vi "标定程序.vi"() -> ()   [LabVIEW 2016]
uses:
  <vilib>/userdefined/High Color/IMAQdx.ctl
  <vilib>/vision/driver/IMAQdx.llb/IMAQdx Acquisition Mode.ctl
  <vilib>/vision/driver/IMAQdx.llb/IMAQdx Buffer Number Mode.ctl
  <vilib>/Utility/config.llb/Read Key (Double).vi
  <vilib>/vision/driver/NI_Vision_Acquisition_Software.lvlib
  <vilib>/Utility/config.llb/NI_LVConfig.lvlib
panel:
  out "Top":cluster{"下边缘设置：":i32, "右边缘设置：":i32}
  out "Bottom":cluster{"上边缘设置：":i32, "右边缘设置：":i32}
  out "CamAng":dbl
  out "RobAng":dbl
  in  "选项卡控件":enum32{"选项卡 1"}(tab)
  out "Image":T1(plugin-control)
  out "机械手参数设置":bool
  out "机械手连接":bool
  out "相机一次采集":bool
  out "机械手X轴移动":bool
  out "相机二次采集":bool
  out "示教圆心":bool
  out "参数保存":bool
  in  "机械手IP地址":string="10.193.13.22"
  in  "机械手端口号":string="54600"
  in  "X轴偏移量":string="10"
  in  "Y轴偏移量":string="10"
  out "机械手Y轴移动":bool
  out "相机三次采集":bool
  in  "Fail步骤":string
  out "机械手当前X坐标":dbl
  out "机械手当前Y坐标":dbl
  out "圆心像素X坐标":dbl
  out "圆心像素Y坐标":dbl
  in  "确定按钮":bool
  in  "强制退出":bool
  out "停止2":bool
  out "停止":bool
  out "数组 2":dbl[](array[numeric])
  out "数组":dbl[](array[numeric])
  out "是否重建模板":bool
  in  "操作状态":string
  out "step8":bool
  out "step7":bool
  out "step6":bool
  out "step5":bool
  out "step4":bool
  out "step3":bool
  out "step2":bool
  out "执行状态":bool
  in  "机械手坐标系":string
  out "step1":bool
  # "库卡机械手视觉标定程序"
  # "V1.0"
  # "机械手参数显示"
  # "视觉影像显示"
  # "位置参数显示"
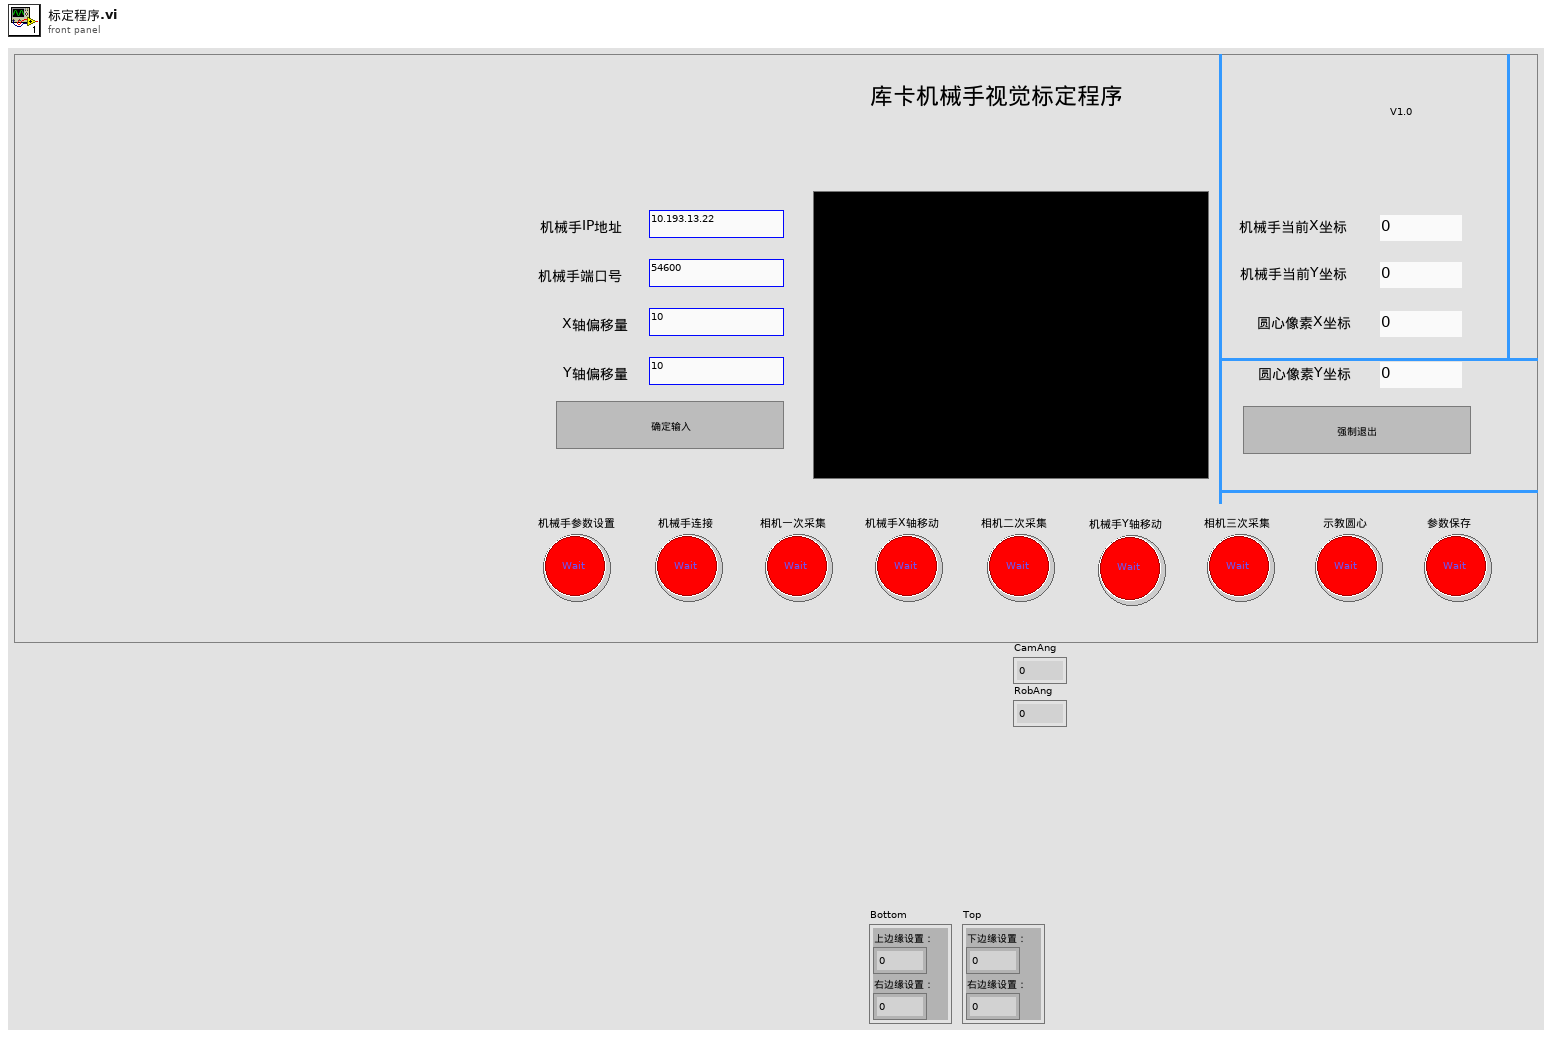
[diagram p1: front panel]
types:
  T1 = typedef "IMAQ Image.ctl" = refnum<image>
  T2 = typedef "NI_Vision_Acquisition_Software.lvlib/IMAQdx Acquisition Mode.ctl" = enum32{"One Shot", "Continuous"}
  T3 = typedef "IMAQdx.ctl" = refnum<k21>
  T4 = enum16{"初始化", "机械手参数设置", "机械手连接", "相机一次采集", "机械手X轴移动", "相机二次采集", "机械手Y轴移动", "相机三次采集", "示教基准位置", "保存参数", "完成"}
  T5 = enum16{"Standard", "Buffered", "CRLF", "Immediate"}
  T6 = typedef "NI_Vision_Acquisition_Software.lvlib/IMAQdx Buffer Number Mode.ctl" = enum32{"Next", "Last", "Buffer Number", "Every", "Last New"}
  T7 = enum32{"Invalid", "Standard", "Closed", "Hidden", "Minimized", "Maximized"}
  T8 = typedef "NI_LVConfig.lvlib/Config Data RefNum.ctl" = refnum<k1>
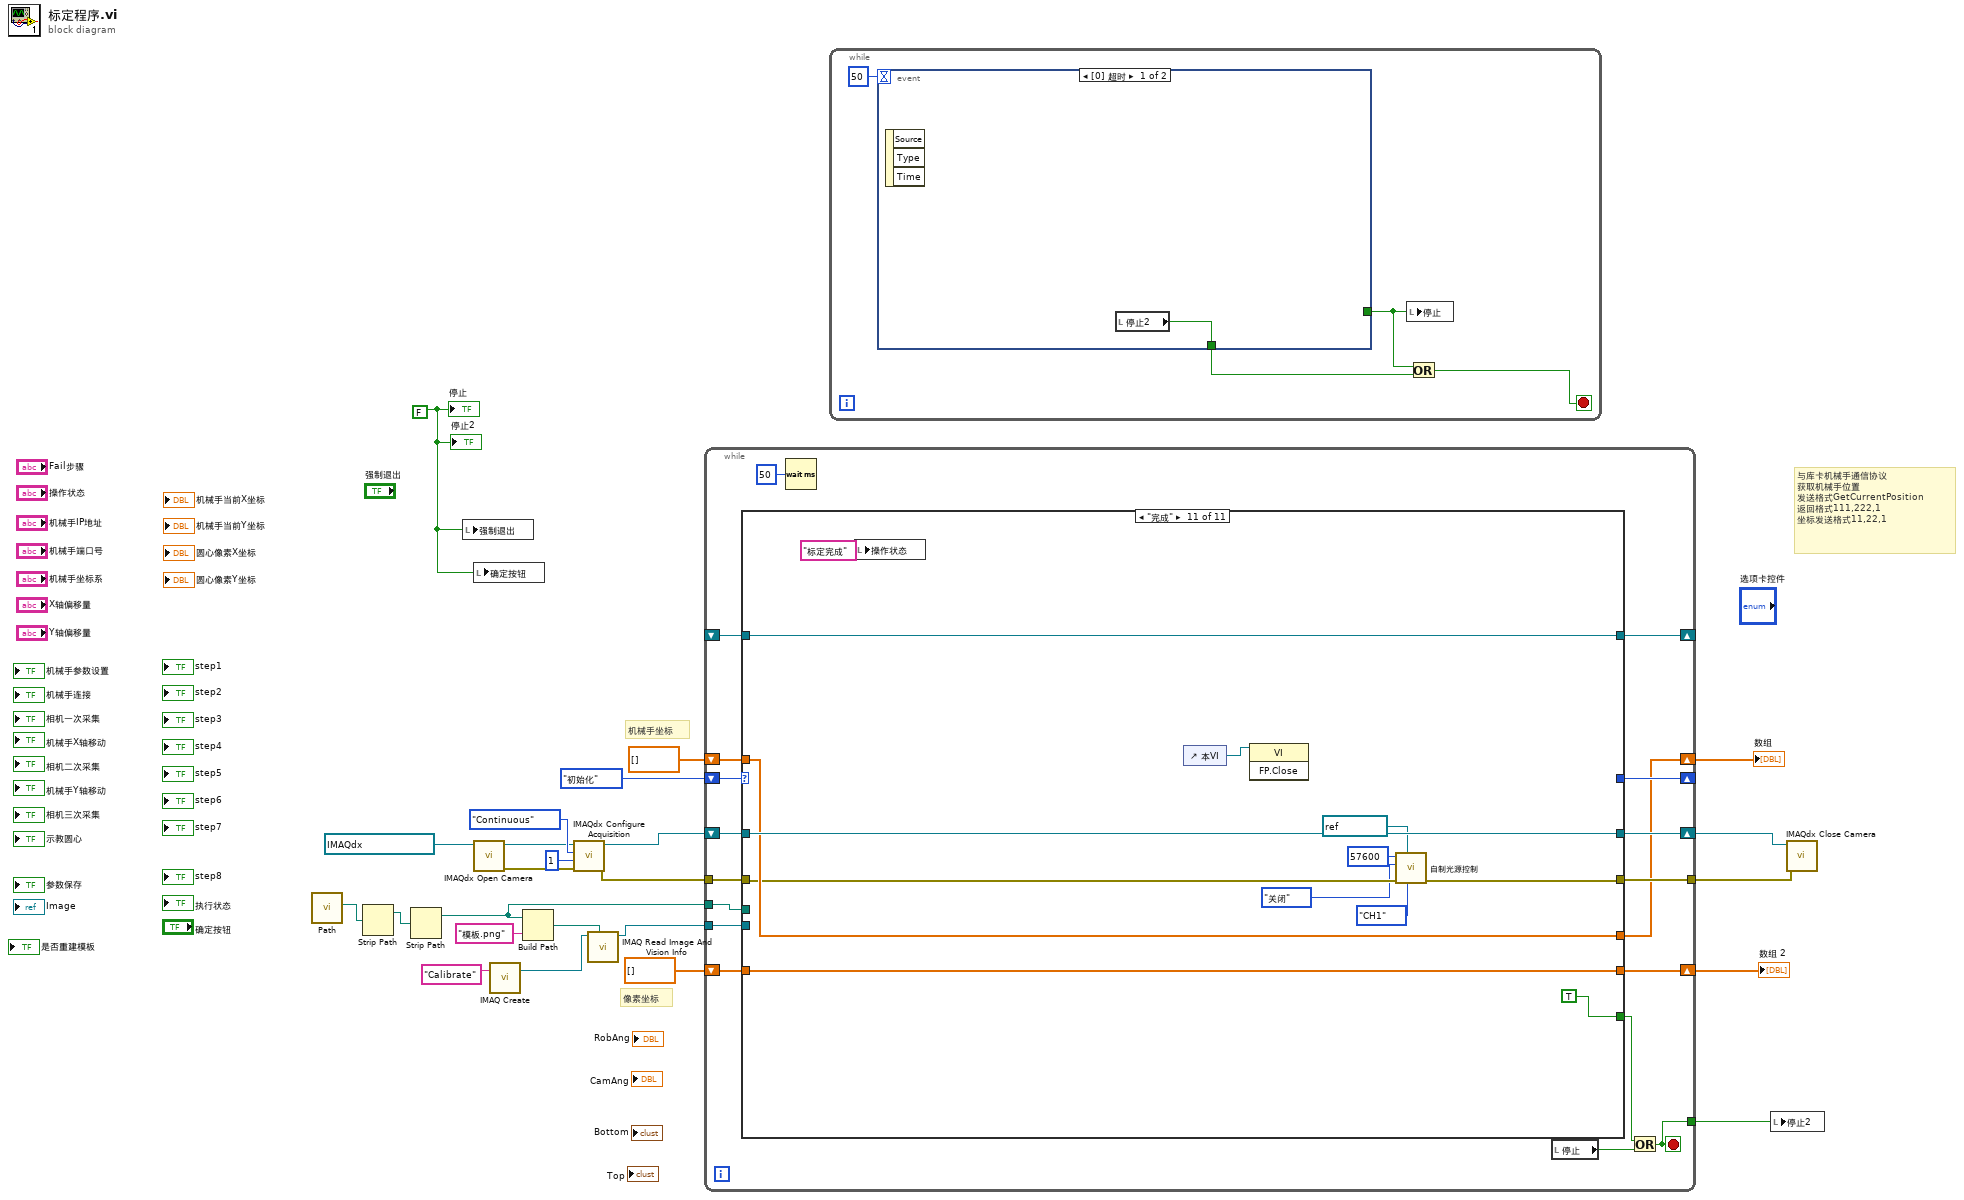
[diagram p0: block diagram]
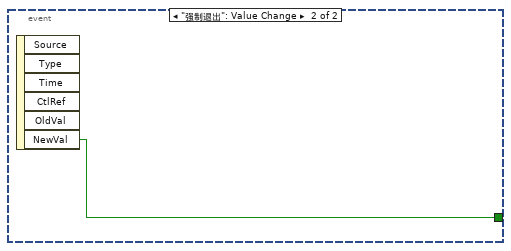
[diagram p2: hidden frame]
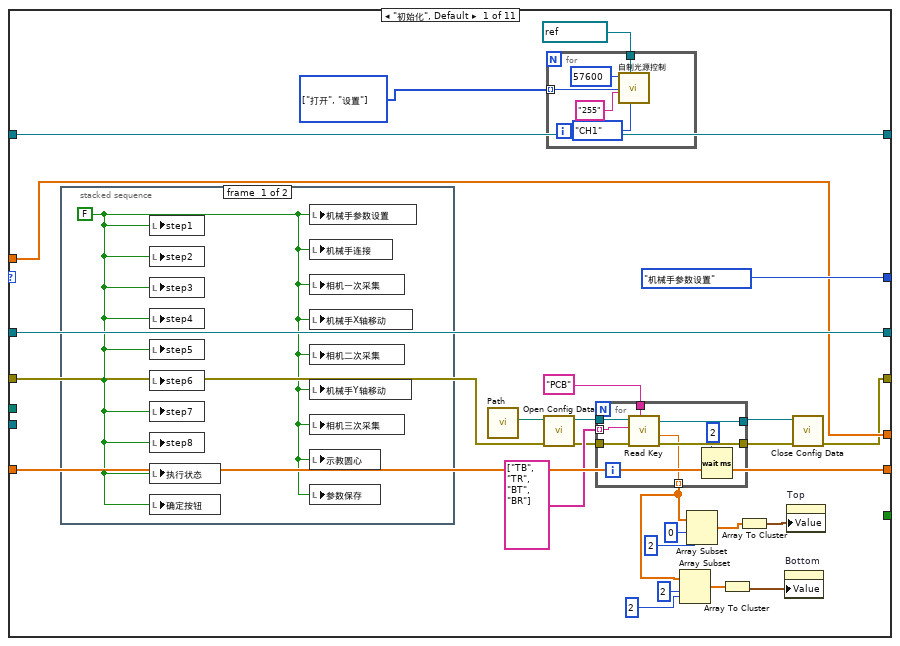
[diagram p3: hidden frame]
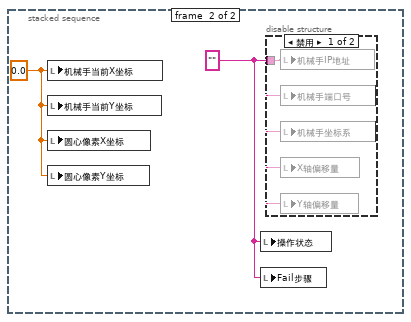
[diagram p4: hidden frame]
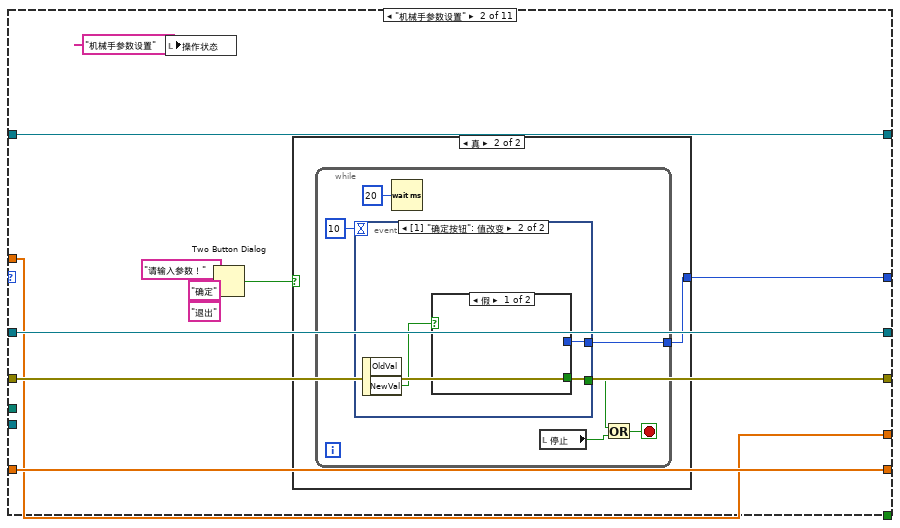
[diagram p6: hidden frame]
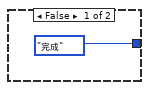
[diagram p7: hidden frame]
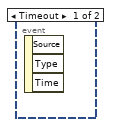
[diagram p8: hidden frame]
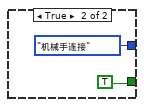
[diagram p9: hidden frame]
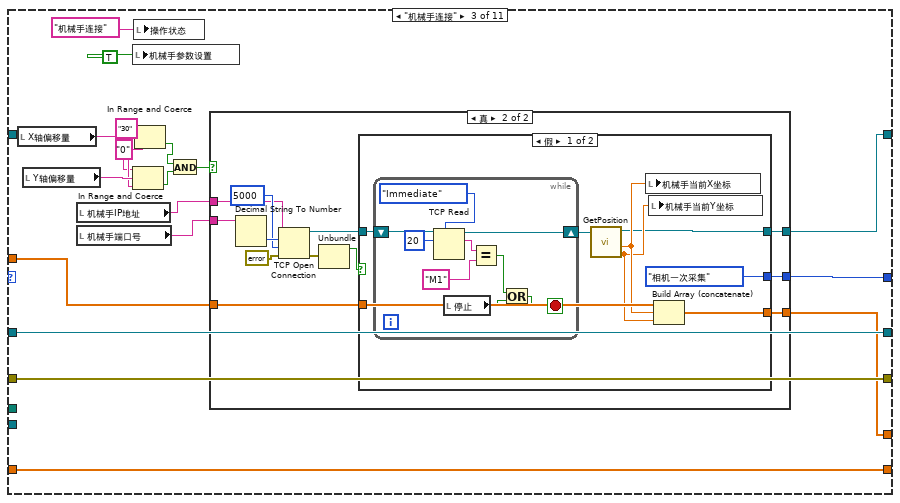
[diagram p10: hidden frame]
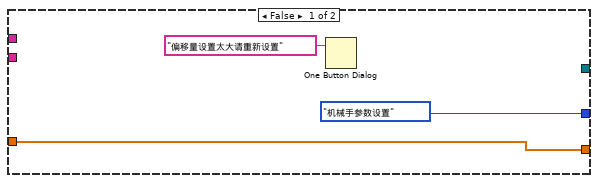
[diagram p11: hidden frame]
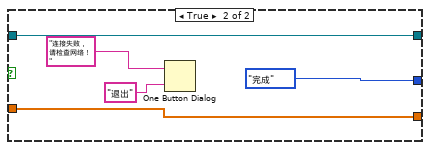
[diagram p12: hidden frame]
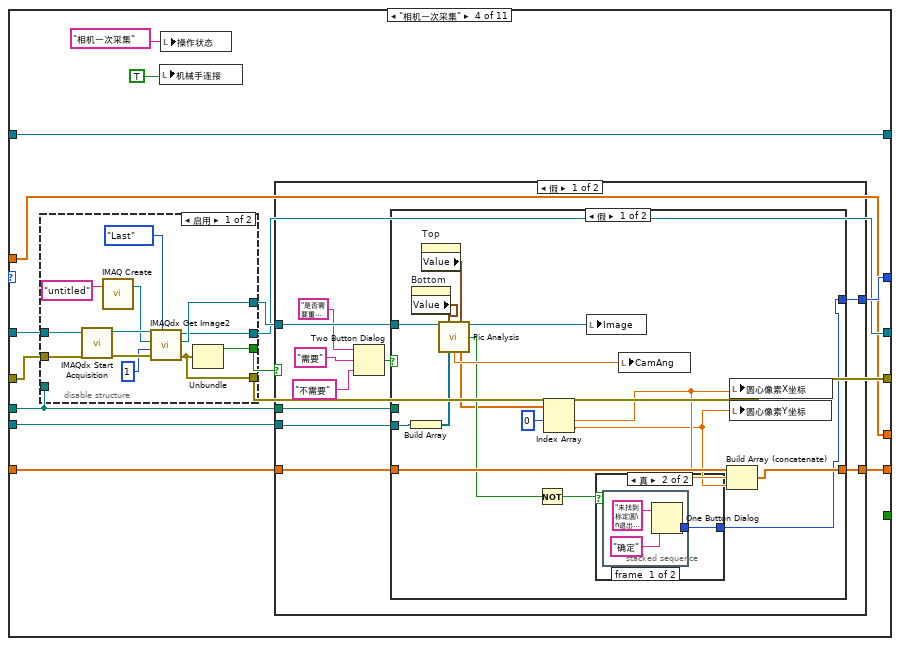
[diagram p13: hidden frame]
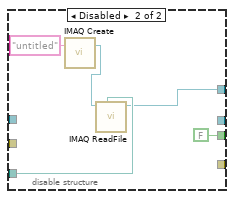
[diagram p14: hidden frame]
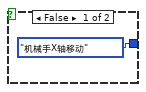
[diagram p15: hidden frame]
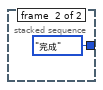
[diagram p16: hidden frame]
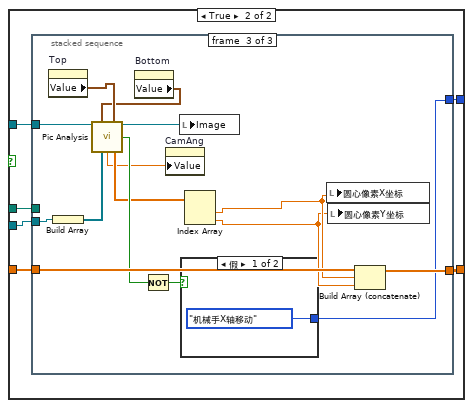
[diagram p17: hidden frame]
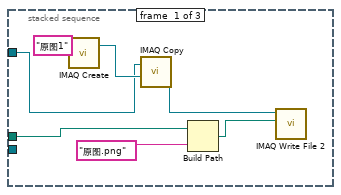
[diagram p18: hidden frame]
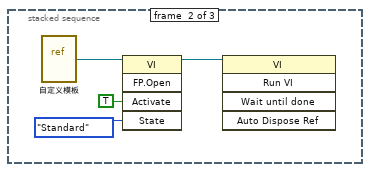
[diagram p19: hidden frame]
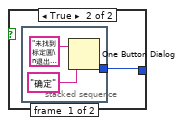
[diagram p20: hidden frame]
diagram:
  w8 = FALSE
  # "与库卡机械手通信协议\n获取机械手位置\n发送格式GetCurrentPosition\n返回格式111,222,1\n坐标发送格式11,22,1"
  # "机械手坐标"
  # "像素坐标"
  n1 = call "Path.vi"() -> ("ini"=w7:path)  [unwired: 11 in]
  n2 = Strip Path(path=w7) -> (stripped path=w6:path)  [unwired: 1 out]
  n3 = Strip Path(path=w6) -> (stripped path=w5:path)  [unwired: 1 out]
  n4 = local write "强制退出"(w8) -> ()
  n5 = local write "确定按钮"(w8) -> ()
  n6 = call <vilib>:"IMAQdx Open Camera.vi"("Session In"=T3 "acA1600-20gc") -> ("error out"=w17:errorcluster, "Session Out"=w21:T3)  [unwired: 9 in]
  n7 = call "IMAQ Create"("Image Name"="Calibrate") -> ("New Image"=w2:T1)  [unwired: 4 in, 1 out]
  n8 = Build Path(base path=w5, name or relative path="模板.png" ("名称或相对路径")) -> (appended path=w4:path)
  n9 = call <vilib>:"IMAQdx Configure Acquisition.vi"("error in"=w17, "Number of Buffers"=u32 1, "Continuous?"=IMAQdx_Acquisition_Mode."Continuous", "Session In"=w21) -> ("error out"=w16:errorcluster, "Session Out"=w19:T3)  [unwired: 6 in]
  n10 = call "IMAQ Read Image And Vision Info"("File Path"=w4, "Image"=w2) -> ("Image Out"=w1:T1)  [unwired: 7 in, 2 out]
  n11 = while {
    shift-right: [w41] -> _
    shift-left: T4."初始化" -> [w42]
    shift-right: [w40] -> _
    shift-left: _ -> [w31]
    shift-right: [w38] -> w18
    shift-left: w19 -> [w39]
    tunnel: w16 -> [w37]
    tunnel: [w36] -> w15
    tunnel: w1 -> [w35]
    shift-right: [w33] -> w10
    shift-left: dbl[] [] -> [w34]
    shift-right: [w28] -> w11
    shift-left: dbl[] [] -> [w32]
    tunnel: w5 -> [w30]
    tunnel: [w25] -> w9
    stop <- w25 stop-if-true
    n12 = case shown="\"完成\"" w42 {
      tunnel: [T4."机械手参数设置" w91 w126 w176 T4."相机二次采集" w304 T4."相机三次采集" w383 w428 T4."完成" _] -> w41
      tunnel: [_ _ _ _ _ _ _ _ _ _ TRUE] -> w27
      tunnel: [w66 w90 w122 w174 w274 w298 _ _ _ w494 w506] -> w40
      tunnel: w39 -> [w65 w89 w125 w178 w283 w306 w361 w385 w436 w493 w505]
      tunnel: [w65 w89 w125 w167 w283 w303 w361 w382 w436 w493 w505] -> w38
      tunnel: w37 -> [w48 w88 w124 w177 w282 w305 w362 w384 w435 w492 w502]
      tunnel: w31 -> [w66 w90 _ w174 w272 w298 w351 _ _ w494 w506]
      tunnel: [w47 w88 w124 w173 w282 w302 w362 w381 w435 w492 w501] -> w36
      tunnel: w35 -> [_ _ _ w171 _ w297 _ w377 _ _ _]
      tunnel: w34 -> [w64 w86 w121 w170 w284 w301 w363 w379 w433 w480 w504]
      tunnel: [w64 w86 w121 w169 w284 w300 w363 w378 w433 w480 w504] -> w33
      tunnel: w32 -> [w63 w85 w120 w165 w279 w296 w359 w376 w432 w484 w503]
      tunnel: w30 -> [_ _ _ w166 _ _ _ _ _ _ _]
      tunnel: [w63 w85 w118 w165 w268 w296 w349 w376 w427 w484 w503] -> w28
      frame "初始化", Default {
        w43 = enum16{"打开", "关闭", "设置"}[] [enum."打开", enum."设置"] items=["打开", "关闭", "设置"]
        n13 = stacked-sequence {
          frame #0 {
            w81 = FALSE ("step1")
            n14 = local write "step1"(w81) -> ()
            n15 = local write "step2"(w81) -> ()
            n16 = local write "step3"(w81) -> ()
            n17 = local write "step4"(w81) -> ()
            n18 = local write "step5"(w81) -> ()
            n19 = local write "step6"(w81) -> ()
            n20 = local write "step7"(w81) -> ()
            n21 = local write "step8"(w81) -> ()
            n22 = local write "执行状态"(w81) -> ()
            n23 = local write "确定按钮"(w81) -> ()
            n24 = local write "机械手参数设置"(w81) -> ()
            n25 = local write "机械手连接"(w81) -> ()
            n26 = local write "相机一次采集"(w81) -> ()
            n27 = local write "机械手X轴移动"(w81) -> ()
            n28 = local write "相机二次采集"(w81) -> ()
            n29 = local write "机械手Y轴移动"(w81) -> ()
            n30 = local write "相机三次采集"(w81) -> ()
            n31 = local write "示教圆心"(w81) -> ()
            n32 = local write "参数保存"(w81) -> ()
          }
          frame #1 {
            w82 = ""
            w83 = 0.0 ("机械手当前X坐标")
            n33 = local write "机械手当前X坐标"(w83) -> ()
            n34 = local write "机械手当前Y坐标"(w83) -> ()
            n35 = local write "圆心像素X坐标"(w83) -> ()
            n36 = local write "圆心像素Y坐标"(w83) -> ()
            n37 = local write "操作状态"(w82) -> ()
            n38 = local write "Fail步骤"(w82) -> ()
            n39 = disable-structure shown="禁用" {
              disable-tunnel: w82 -> [w84 _]
              frame Disabled {
                n40 = local write "机械手IP地址"(w84) -> ()
                n41 = local write "机械手端口号"(w84) -> ()
                n42 = local write "机械手坐标系"(w84) -> ()
                n43 = local write "X轴偏移量"(w84) -> ()
                n44 = local write "Y轴偏移量"(w84) -> ()
              }
              frame Enabled {
              }
            }
          }
        }
        n45 = call "Path.vi"() -> ("ini"=w59:path)  [unwired: 11 in]
        n46 = call <vilib>:"Open Config Data.vi"("error in (no error)"=w48, "configuration file path"=w59) -> ("error out"=w50:errorcluster, "refnum"=w49:T8)  [unwired: 7 in, 1 out]
        n47 = for {
          tunnel: refnum<visa-resource-name> "COM1" ("VISA In") -> [w72]
          tunnel: w43 -> [w70] mode=indexing
          n48 = call "自制光源控制.vi"("通道"=enum16{"CH1", "CH2", "CH3", "CH4"}."CH1", "VISA In"=w72, "亮度"="255", "操作模式"=w70, "baud rate"=u32 57600) -> ()  [unwired: 4 in, 3 out]
        }
        n49 = for {
          tunnel: w49 -> [w80]
          tunnel: w50 -> [w79]
          tunnel: "PCB" ("机种") -> [w78]
          tunnel: string[] ["TB", "TR", "BT", "BR"] -> [w77] mode=indexing
          tunnel: [w76] -> w62
          tunnel: [w75] -> w61
          tunnel: [w74] -> w58 mode=indexing
          n50 = call-poly <vilib>:"Read Key.vi"("section"=w78, "error in (no error)"=w79, "key"=w77, "refnum"=w80) -> ("error out"=w75:errorcluster, "value"=w74:dbl, "refnum out"=w76:T8)  [unwired: 4 in, 1 out]
          n51 = Wait (ms)(milliseconds to wait=u32 2 ("等待时间（毫秒）")) -> ()  [unwired: 1 out]
        }
        n52 = Array Subset(array=w58, index=2 ("索引"), length=2 ("长度")) -> (w57:dbl[])
        n53 = Array Subset(array=w58, index=0 ("索引"), length=2 ("长度")) -> (w54:dbl[])
        n54 = Array To Cluster(array=w57) -> (cluster=w45:cluster{"[0]":dbl, "[1]":dbl})
        n55 = Array To Cluster(array=w54) -> (cluster=w46:cluster{"[0]":dbl, "[1]":dbl})
        n56 = property on="Bottom" class="Clust (严格)"("Value"=w45) -> ()  [unwired: 2 in, 2 out]
        n57 = property on="Top" class="Clust (严格)"("Value"=w46) -> ()  [unwired: 2 in, 2 out]
        n58 = call <vilib>:"Close Config Data.vi"("error in (no error)"=w61, "refnum"=w62) -> ("error out"=w47:errorcluster)  [unwired: 8 in, 1 out]
      }
      frame "机械手参数设置" {
        n59 = local write "操作状态"("机械手参数设置" ("操作状态")) -> ()
        n60 = Two Button Dialog(message="请输入参数！" ("消息"), 1:"退出" ("按钮名称（“确定”）"), 2:"确定" ("T按钮名称（“确定”）")) -> (T button?=w92:bool)
        n61 = case shown="真" w92 {
          tunnel: [T4."完成" w97] -> w91
          frame False {
          }
          frame True {
            n62 = while {
              tunnel: [w103] -> w97
              stop <- w98 stop-if-true
              n63 = event shown="[1] \"确定按钮\": 值改变" {
                selector: _ -> [_ _]
                dyn-events: _ -> [_ _]
                timeout: 10 -> [_ _]
                tunnel: [_ w105] -> w99
                tunnel: [_ w104] -> w103
                event Timeout {
                  n64 = event-data() -> ()  [unwired: 1 in, 3 out]
                }
                event "确定按钮": Value Change {
                  n65 = event-data() -> ("NewVal"=w106:bool)  [unwired: 1 in, 1 out]
                  n66 = case shown="假" w106 {
                    tunnel: [_ TRUE] -> w105
                    tunnel: [_ T4."机械手连接"] -> w104
                    frame False {
                    }
                    frame True {
                    }
                  }
                }
              }
              n67 = Wait (ms)(milliseconds to wait=u32 20 ("等待时间（毫秒）")) -> ()  [unwired: 1 out]
              n68 = local read "停止"() -> (w100:bool)
              n69 = Or(x=w99, y=w100) -> (x .or. y?=w98:bool)
            }
          }
        }
      }
      frame "机械手连接" {
        w112 = "0" ("下限")
        w111 = "30" ("上限")
        n70 = local read "X轴偏移量"() -> (w117:string)
        n71 = local read "Y轴偏移量"() -> (w116:string)
        n72 = local read "机械手IP地址"() -> (w110:string)
        n73 = local read "机械手端口号"() -> (w109:string)
        n74 = local write "机械手参数设置"(TRUE ("机械手参数设置")) -> ()
        n75 = In Range and Coerce(upper limit=w111, x=w116, lower limit=w112) -> (In Range?=w114:bool)  [unwired: 1 out]
        n76 = local write "操作状态"("机械手连接" ("操作状态")) -> ()
        n77 = In Range and Coerce(upper limit=w111, x=w117, lower limit=w112) -> (In Range?=w115:bool)  [unwired: 1 out]
        n78 = And(x=w115, y=w114) -> (x .and. y?=w113:bool)
        n79 = case shown="真" w113 {
          tunnel: [T4."机械手参数设置" w137] -> w126
          tunnel: [_ w134] -> w122
          tunnel: w120 -> [w128 w133]
          tunnel: [w128 w132] -> w118
          tunnel: w110 -> [_ w131]
          tunnel: w109 -> [_ w130]
          frame False {
            n80 = One Button Dialog(message="偏移量设置太大请重新设置" ("消息")) -> ()  [unwired: 1 in, 1 out]
          }
          frame True {
            n81 = Decimal String To Number(string=w130) -> (number=w141:i32)  [unwired: 2 in, 1 out]
            n82 = TCP Open Connection(address=w131, remote port or service name=w141, timeout ms (60000)=5000 ("超时毫秒(60000)"), error in (no error)=errorcluster {"status"=FALSE, "code"=0, "source"=""} ("错误输入（无错误）")) -> (connection ID=w135:refnum<k5>, error out=w139:errorcluster)  [unwired: 1 in]
            n83 = Unbundle(w139) -> ("status"=w138:bool)  [unwired: 2 out]
            n84 = case shown="假" w138 {
              tunnel: [T4."相机一次采集" T4."完成"] -> w137
              tunnel: w135 -> [w143 w162]
              tunnel: [w144 w162] -> w134
              tunnel: w133 -> [w148 w161]
              tunnel: [w147 w161] -> w132
              frame False {
                n85 = while {
                  shift-right: [w156] -> w142
                  shift-left: w143 -> [w158]
                  stop <- w151 stop-if-true
                  n86 = TCP Read(connection ID=w158, bytes to read=20 ("读取的字节"), 7:T5."Immediate" ("模式（标准）")) -> (connection ID out=w156:refnum<k5>, data out=w155:string)  [unwired: 2 in, 1 out]
                  n87 = local read "停止"() -> (w150:bool)
                  n88 = Equal?(x=w155, y="M1") -> (x = y?=w152:bool)
                  n89 = Or(x=w152, y=w150) -> (x .or. y?=w151:bool)
                }
                n90 = call "GetPosition.vi"("连接ID"=w142) -> ("y"=w145:dbl, "x"=w146:dbl, "连接ID 2"=w144:refnum<k5>)  [unwired: 5 in, 1 out]
                n91 = local write "机械手当前X坐标"(w146) -> ()
                n92 = local write "机械手当前Y坐标"(w145) -> ()
                n93 = Build Array (concatenate)(w148, w146, w145) -> (w147:dbl[])
              }
              frame True {
                n94 = One Button Dialog(message="连接失败，请检查网络！" ("消息"), button name ("OK")="退出" ("按钮名称（“确定”）")) -> ()  [unwired: 1 out]
              }
            }
          }
        }
      }
      frame "相机一次采集" {
        n95 = disable-structure shown="启用" {
          disable-tunnel: w178 -> [w187 _]
          disable-tunnel: w177 -> [w186 _]
          disable-tunnel: [w182 FALSE ("status")] -> w164
          disable-tunnel: [w181 w191] -> w175
          disable-tunnel: [w180 _] -> w173
          disable-tunnel: [w179 _] -> w167
          disable-tunnel: w166 -> [_ w192]
          frame Enabled {
            n96 = call <vilib>:"IMAQdx Start Acquisition.vi"("error in"=w186, "Session In"=w187) -> ("error out"=w185:errorcluster, "Session Out"=w190:T3)  [unwired: 8 in]
            n97 = call "IMAQ Create"("Image Name"="untitled") -> ("New Image"=w189:T1)  [unwired: 4 in, 1 out]
            n98 = call <vilib>:"IMAQdx Get Image2.vi"("Buffer Number Mode (Next)"=IMAQdx_Buffer_Number_Mode."Last", "error in"=w185, "Buffer Number In"=u32 1, "Image In"=w189, "Session In"=w190) -> ("error out"=w180:errorcluster, "Image Out"=w181:T1, "Session Out"=w179:T3)  [unwired: 3 in, 1 out]
            n99 = Unbundle(w180) -> ("status"=w182:bool)  [unwired: 2 out]
          }
          frame Disabled {
            n100 = call "IMAQ Create"("Image Name"="untitled") -> ("New Image"=w193:T1)  [unwired: 4 in, 1 out]
            n101 = call "IMAQ ReadFile"("File Path"=w192, "Image"=w193) -> ("Image Out"=w191:T1)  [unwired: 5 in, 4 out]
          }
        }
        n102 = local write "机械手连接"(TRUE ("机械手参数设置")) -> ()
        n103 = local write "操作状态"("相机一次采集" ("操作状态")) -> ()
        n104 = case shown="假" w164 {
          tunnel: [w205 T4."完成"] -> w176
          tunnel: w175 -> [w204 _]
          tunnel: w171 -> [w199 _]
          tunnel: w170 -> [w198 w266]
          tunnel: [w197 w266] -> w169
          tunnel: w166 -> [w196 _]
          frame False {
            n105 = Two Button Dialog(message="是否需要重新定义模板？" ("消息"), 1:"不需要" ("F按钮名称（“取消”）"), 2:"需要" ("T按钮名称（“确定”）")) -> (T button?=w200:bool)
            n106 = case shown="假" w200 {
              tunnel: [w219 w231] -> w205
              tunnel: w204 -> [w218 w232]
              tunnel: w199 -> [w216 w230]
              tunnel: w198 -> [w221 w229]
              tunnel: [w220 w228] -> w197
              tunnel: w196 -> [_ w227]
              frame False {
                n107 = Build Array(w216) -> (w215:T1[])
                n108 = property on="Bottom" class="Clust (严格)"() -> ("Value"=w206:cluster{"上边缘设置：":i32, "右边缘设置：":i32})  [unwired: 2 in, 2 out]
                n109 = property on="Top" class="Clust (严格)"() -> ("Value"=w207:cluster{"下边缘设置：":i32, "右边缘设置：":i32})  [unwired: 2 in, 2 out]
                n110 = call "Pic Analysis.vi"("Image in"=w218, "Bottom"=w206, "Top"=w207, "Temp"=w215) -> ("Image"=w217:T1, "Found"=w213:bool, "Angle"=w214:sgl, "Position"=w211:sgl[])  [unwired: 6 in, 2 out]
                n111 = Not(x=w213) -> (.not. x?=w212:bool)
                n112 = Index Array(array=w211, index #1=0 ("索引")) -> (element #1=w209:sgl, element #2=w208:sgl)  [unwired: 1 in]
                n113 = local write "Image"(w217) -> ()
                n114 = case shown="真" w212 {
                  tunnel: [T4."机械手X轴移动" w223] -> w219
                  frame False {
                  }
                  frame True {
                    n115 = stacked-sequence {
                      tunnel: [_ T4."完成"] -> w223
                      frame #0 {
                        n116 = One Button Dialog(message="未找到标定圆\n退出标定重新开始！" ("消息"), button name ("OK")="确定" ("按钮名称（“确定”）")) -> ()  [unwired: 1 out]
                      }
                      frame #1 {
                      }
                    }
                  }
                }
                n117 = local write "CamAng"(w214) -> ()
                n118 = Build Array (concatenate)(w221, w209, w208) -> (w220:dbl[])
                n119 = local write "圆心像素X坐标"(w209) -> ()
                n120 = local write "圆心像素Y坐标"(w208) -> ()
              }
              frame True {
                n121 = stacked-sequence {
                  tunnel: w232 -> [w234 _ w255]
                  tunnel: [_ _ w256] -> w231
                  tunnel: w230 -> [_ _ w253]
                  tunnel: w229 -> [_ _ w258]
                  tunnel: [_ _ w257] -> w228
                  tunnel: w227 -> [w238 _ _]
                  frame #0 {
                    n122 = call "IMAQ Create"("Image Name"="原图1") -> ("New Image"=w235:T1)  [unwired: 4 in, 1 out]
                    n123 = call "IMAQ Copy"("Image Dst"=w235, "Image Src"=w234) -> ("Image Dst Out"=w233:T1)  [unwired: 4 in, 1 out]
                    n124 = Build Path(base path=w238, name or relative path="原图.png" ("字符串")) -> (appended path=w239:path)
                    n125 = call-poly "IMAQ Write File 2"("File Path"=w239, "Image"=w233) -> ()  [unwired: 8 in, 2 out]
                  }
                  frame #1 {
                    n126 = vi-ref "自定义模板.vi"() -> (w243:refnum<vi>)
                    n127 = invoke class="VI" method="FP.Open"(reference=w243, "Activate"=TRUE ("激活？"), "State"=T7."Standard" ("状态")) -> (reference out=w240:refnum<vi>)  [unwired: 2 in, 4 out]
                    n128 = invoke class="VI" method="Run VI"(reference=w240) -> ()  [unwired: 4 in, 5 out]
                  }
                  frame #2 {
                    n129 = property on="Top" class="Clust (严格)"() -> ("Value"=w246:cluster{"下边缘设置：":i32, "右边缘设置：":i32})  [unwired: 2 in, 2 out]
                    n130 = Build Array(w253) -> (w252:T1[])
                    n131 = property on="Bottom" class="Clust (严格)"() -> ("Value"=w245:cluster{"上边缘设置：":i32, "右边缘设置：":i32})  [unwired: 2 in, 2 out]
                    n132 = call "Pic Analysis.vi"("Image in"=w255, "Bottom"=w245, "Top"=w246, "Temp"=w252) -> ("Image"=w254:T1, "Found"=w250:bool, "Angle"=w244:sgl, "Position"=w249:sgl[])  [unwired: 6 in, 2 out]
                    n133 = Not(x=w250) -> (.not. x?=w251:bool)
                    n134 = property on="CamAng" class="DigNum (严格)"("Value"=w244) -> ()  [unwired: 2 in, 2 out]
                    n135 = local write "Image"(w254) -> ()
                    n136 = case shown="假" w251 {
                      tunnel: [T4."机械手X轴移动" w260] -> w256
                      frame False {
                      }
                      frame True {
                        n137 = stacked-sequence {
                          tunnel: [_ T4."完成"] -> w260
                          frame #0 {
                            n138 = One Button Dialog(message="未找到标定圆\n退出标定重新开始！" ("消息"), button name ("OK")="确定" ("按钮名称（“确定”）")) -> ()  [unwired: 1 out]
                          }
                          frame #1 {
                          }
                        }
                      }
                    }
                    n139 = Index Array(array=w249) -> (element #1=w248:sgl, element #2=w247:sgl)  [unwired: 2 in]
                    n140 = local write "圆心像素X坐标"(w248) -> ()
                    n141 = local write "圆心像素Y坐标"(w247) -> ()
                    n142 = Build Array (concatenate)(w258, w248, w247) -> (w257:dbl[])
                  }
                }
              }
            }
          }
          frame True {
            n143 = One Button Dialog(message="相机出错，检查相机连接！" ("消息"), button name ("OK")="确定" ("按钮名称（“确定”）")) -> ()  [unwired: 1 out]
          }
        }
      }
      frame "机械手X轴移动" {
        n144 = local read "机械手当前X坐标"() -> (w277:dbl)
        n145 = local read "机械手当前Y坐标"() -> (w275:dbl)
        n146 = local write "操作状态"("机械手X轴移动" ("操作状态")) -> ()
        n147 = local write "相机一次采集"(TRUE ("机械手参数设置")) -> ()
        n148 = local read "X轴偏移量"() -> (w273:string)
        n149 = Decimal String To Number(string=w273) -> (number=w278:i32)  [unwired: 2 in, 1 out]
        n150 = call "发送指令.vi"("X"=w273) -> ("发送指令"=w271:string)  [unwired: 4 in]
        n151 = Add(x=w278, y=w277) -> (x+y=w276:dbl)
        n152 = TCP Write(connection ID=w272, data in=w271, 9:3000 ("超时毫秒(25000)")) -> (connection ID out=w270:refnum<k5>)  [unwired: 1 in, 2 out]
        n153 = while {
          shift-right: [w293] -> w274
          shift-left: w270 -> [w289]
          stop <- w286 stop-if-true
          n154 = TCP Read(connection ID=w289, bytes to read=512 ("读取的字节"), 7:T5."Immediate" ("模式（标准）"), 9:200 ("超时毫秒(25000)")) -> (connection ID out=w293:refnum<k5>, data out=w291:string)  [unwired: 1 in, 1 out]
          n155 = local read "停止"() -> (w287:bool)
          n156 = Equal?(x=w291, y="ok") -> (x = y?=w288:bool)
          n157 = Or(x=w288, y=w287) -> (x .or. y?=w286:bool)
        }
        n158 = Build Array (concatenate)(w279, w276, w275) -> (w268:dbl[])
        n159 = local write "机械手当前X坐标"(w276) -> ()
        n160 = local write "机械手当前Y坐标"(w275) -> ()
      }
      frame "相机二次采集" {
        n161 = disable-structure shown="启用" {
          disable-tunnel: [w315 FALSE ("status")] -> w308
          disable-tunnel: [w314 w323] -> w307
          disable-tunnel: w306 -> [w313 _]
          disable-tunnel: w305 -> [w312 _]
          disable-tunnel: [w311 _] -> w303
          disable-tunnel: [w310 _] -> w302
          disable-tunnel: w297 -> [_ w322]
          frame Enabled {
            n162 = call <vilib>:"IMAQdx Start Acquisition.vi"("error in"=w312, "Session In"=w313) -> ("error out"=w318:errorcluster, "Session Out"=w321:T3)  [unwired: 8 in]
            n163 = call "IMAQ Create"("Image Name"="untitled") -> ("New Image"=w320:T1)  [unwired: 4 in, 1 out]
            n164 = call <vilib>:"IMAQdx Get Image2.vi"("Buffer Number Mode (Next)"=IMAQdx_Buffer_Number_Mode."Last", "error in"=w318, "Buffer Number In"=u32 1, "Image In"=w320, "Session In"=w321) -> ("error out"=w310:errorcluster, "Image Out"=w314:T1, "Session Out"=w311:T3)  [unwired: 3 in, 1 out]
            n165 = Unbundle(w310) -> ("status"=w315:bool)  [unwired: 2 out]
          }
          frame Disabled {
            n166 = call "IMAQ Create"("Image Name"="untitled") -> ("New Image"=w324:T1)  [unwired: 4 in, 1 out]
            n167 = call "IMAQ ReadFile"("File Path"=w322, "Image"=w324) -> ("Image Out"=w323:T1)  [unwired: 5 in, 4 out]
          }
        }
        n168 = local write "机械手X轴移动"(TRUE ("机械手参数设置")) -> ()
        n169 = local write "操作状态"("相机二次采集" ("操作状态")) -> ()
        n170 = case shown="假" w308 {
          tunnel: [w339 T4."完成"] -> w304
          tunnel: w307 -> [w338 _]
          tunnel: w297 -> [w336 _]
          tunnel: w301 -> [w341 w346]
          tunnel: [w340 w346] -> w300
          frame False {
            n171 = property on="Bottom" class="Clust (严格)"() -> ("Value"=w327:cluster{"上边缘设置：":i32, "右边缘设置：":i32})  [unwired: 2 in, 2 out]
            n172 = property on="Top" class="Clust (严格)"() -> ("Value"=w328:cluster{"下边缘设置：":i32, "右边缘设置：":i32})  [unwired: 2 in, 2 out]
            n173 = Build Array(w336) -> (w335:T1[])
            n174 = call "Pic Analysis.vi"("Image in"=w338, "Bottom"=w327, "Top"=w328, "Temp"=w335) -> ("Image"=w337:T1, "Found"=w334:bool, "Position"=w332:sgl[])  [unwired: 6 in, 3 out]
            n175 = local write "Image"(w337) -> ()
            n176 = Index Array(array=w332, index #1=0 ("索引")) -> (element #1=w330:sgl, element #2=w329:sgl)  [unwired: 1 in]
            n177 = Not(x=w334) -> (.not. x?=w333:bool)
            n178 = case shown="真" w333 {
              tunnel: [T4."机械手Y轴移动" T4."完成"] -> w339
              frame False {
              }
              frame True {
                n179 = stacked-sequence {
                  frame #0 {
                    n180 = One Button Dialog(message="未找到标定圆\n退出标定重新开始！" ("消息"), button name ("OK")="确定" ("按钮名称（“确定”）")) -> ()  [unwired: 1 out]
                  }
                  frame #1 {
                  }
                }
              }
            }
            n181 = local write "圆心像素X坐标"(w330) -> ()
            n182 = local write "圆心像素Y坐标"(w329) -> ()
            n183 = Build Array (concatenate)(w341, w330, w329) -> (w340:dbl[])
          }
          frame True {
          }
        }
      }
      frame "机械手Y轴移动" {
        n184 = local read "机械手当前X坐标"() -> (w356:dbl)
        n185 = local read "机械手当前Y坐标"() -> (w357:dbl)
        n186 = local read "Y轴偏移量"() -> (w354:string)
        n187 = local write "相机二次采集"(TRUE ("机械手参数设置")) -> ()
        n188 = local write "操作状态"("机械手Y轴移动" ("操作状态")) -> ()
        n189 = Decimal String To Number(string=w354) -> (number=w358:i32)  [unwired: 2 in, 1 out]
        n190 = call "发送指令.vi"("Y"=w354) -> ("发送指令"=w352:string)  [unwired: 4 in]
        n191 = Add(x=w358, y=w357) -> (x+y=w355:dbl)
        n192 = TCP Write(connection ID=w351, data in=w352, 9:2000 ("超时毫秒(25000)")) -> (connection ID out=w350:refnum<k5>)  [unwired: 1 in, 2 out]
        n193 = while {
          shift-right: [w373] -> w348
          shift-left: w350 -> [w370]
          stop <- w366 stop-if-true
          n194 = TCP Read(connection ID=w370, bytes to read=512 ("读取的字节"), 7:T5."Immediate" ("模式（标准）"), 9:200 ("超时毫秒(25000)")) -> (connection ID out=w373:refnum<k5>, data out=w371:string)  [unwired: 1 in, 1 out]
          n195 = local read "停止"() -> (w367:bool)
          n196 = Equal?(x=w371, y="ok") -> (x = y?=w368:bool)
          n197 = Or(x=w368, y=w367) -> (x .or. y?=w366:bool)
        }
        n198 = Build Array (concatenate)(w359, w356, w355) -> (w349:dbl[])
        n199 = local write "机械手当前X坐标"(w356) -> ()
        n200 = local write "机械手当前Y坐标"(w355) -> ()
        n201 = TCP Read(connection ID=w348) -> ()  [unwired: 4 in, 3 out]
      }
      frame "相机三次采集" {
        n202 = disable-structure shown="启用" {
          disable-tunnel: [w394 FALSE ("status")] -> w387
          disable-tunnel: [w393 w402] -> w386
          disable-tunnel: w385 -> [w392 _]
          disable-tunnel: w384 -> [w391 _]
          disable-tunnel: [w390 _] -> w382
          disable-tunnel: [w389 _] -> w381
          disable-tunnel: w377 -> [_ w401]
          frame Enabled {
            n203 = call <vilib>:"IMAQdx Start Acquisition.vi"("error in"=w391, "Session In"=w392) -> ("error out"=w397:errorcluster, "Session Out"=w400:T3)  [unwired: 8 in]
            n204 = call "IMAQ Create"("Image Name"="untitled") -> ("New Image"=w399:T1)  [unwired: 4 in, 1 out]
            n205 = call <vilib>:"IMAQdx Get Image2.vi"("Buffer Number Mode (Next)"=IMAQdx_Buffer_Number_Mode."Last", "error in"=w397, "Buffer Number In"=u32 1, "Image In"=w399, "Session In"=w400) -> ("error out"=w389:errorcluster, "Image Out"=w393:T1, "Session Out"=w390:T3)  [unwired: 3 in, 1 out]
            n206 = Unbundle(w389) -> ("status"=w394:bool)  [unwired: 2 out]
          }
          frame Disabled {
            n207 = call "IMAQ Create"("Image Name"="untitled") -> ("New Image"=w404:T1)  [unwired: 4 in, 1 out]
            n208 = call "IMAQ ReadFile"("File Path"=w401, "Image"=w404) -> ("Image Out"=w402:T1)  [unwired: 5 in, 4 out]
          }
        }
        n209 = local write "操作状态"("相机三次采集" ("操作状态")) -> ()
        n210 = local write "机械手Y轴移动"(TRUE ("机械手参数设置")) -> ()
        n211 = case shown="假" w387 {
          tunnel: [w418 T4."完成"] -> w383
          tunnel: w386 -> [w417 _]
          tunnel: w377 -> [w415 _]
          tunnel: w379 -> [w420 w425]
          tunnel: [w419 w425] -> w378
          frame False {
            n212 = property on="Bottom" class="Clust (严格)"() -> ("Value"=w406:cluster{"上边缘设置：":i32, "右边缘设置：":i32})  [unwired: 2 in, 2 out]
            n213 = Build Array(w415) -> (w414:T1[])
            n214 = property on="Top" class="Clust (严格)"() -> ("Value"=w407:cluster{"下边缘设置：":i32, "右边缘设置：":i32})  [unwired: 2 in, 2 out]
            n215 = call "Pic Analysis.vi"("Image in"=w417, "Bottom"=w406, "Top"=w407, "Temp"=w414) -> ("Image"=w416:T1, "Found"=w412:bool, "Position"=w411:sgl[])  [unwired: 6 in, 3 out]
            n216 = local write "Image"(w416) -> ()
            n217 = Index Array(array=w411, index #1=0 ("索引")) -> (element #1=w409:sgl, element #2=w408:sgl)  [unwired: 1 in]
            n218 = Not(x=w412) -> (.not. x?=w413:bool)
            n219 = case shown="真" w413 {
              tunnel: [T4."示教基准位置" T4."完成"] -> w418
              frame False {
              }
              frame True {
                n220 = stacked-sequence {
                  frame #0 {
                    n221 = One Button Dialog(message="未找到标定圆\n退出标定重新开始！" ("消息"), button name ("OK")="确定" ("按钮名称（“确定”）")) -> ()  [unwired: 1 out]
                  }
                  frame #1 {
                  }
                }
              }
            }
            n222 = local write "圆心像素X坐标"(w409) -> ()
            n223 = local write "圆心像素Y坐标"(w408) -> ()
            n224 = Build Array (concatenate)(w420, w409, w408) -> (w419:dbl[])
          }
          frame True {
          }
        }
      }
      frame "示教基准位置" {
        n225 = One Button Dialog(message="示教基准位置！" ("消息"), button name ("OK")="记录位置" ("按钮名称（“确定”）")) -> (true=w429:bool)
        n226 = case shown="真" w429 {
          tunnel: w432 -> [w439 w442]
          tunnel: [w439 w441] -> w427
          tunnel: [T4."完成" w440] -> w428
          frame False {
          }
          frame True {
            n227 = local read "机械手端口号"() -> (w445:string)
            n228 = local read "机械手IP地址"() -> (w446:string)
            n229 = Decimal String To Number(string=w445) -> (number=w450:i32)  [unwired: 2 in, 1 out]
            n230 = TCP Open Connection(address=w446, remote port or service name=w450, timeout ms (60000)=5000 ("超时毫秒(60000)"), error in (no error)=errorcluster {"status"=FALSE, "code"=0, "source"=""} ("错误输入（无错误）")) -> (connection ID=w443:refnum<k5>, error out=w448:errorcluster)  [unwired: 1 in]
            n231 = Unbundle(w448) -> ("status"=w444:bool)  [unwired: 2 out]
            n232 = case shown="假" w444 {
              tunnel: w443 -> [w458 _]
              tunnel: w442 -> [w456 w469]
              tunnel: [w453 w469] -> w441
              tunnel: [T4."保存参数" T4."完成"] -> w440
              frame False {
                n233 = while {
                  shift-right: [w466] -> w459
                  shift-left: w458 -> [w468]
                  stop <- w460 stop-if-true
                  n234 = TCP Read(connection ID=w468, bytes to read=512 ("读取的字节"), 7:T5."Immediate" ("模式（标准）")) -> (connection ID out=w466:refnum<k5>, data out=w465:string)  [unwired: 2 in, 1 out]
                  n235 = local read "停止"() -> (w461:bool)
                  n236 = Equal?(x=w465, y="M1") -> (x = y?=w462:bool)
                  n237 = Or(x=w462, y=w461) -> (x .or. y?=w460:bool)
                }
                n238 = call "GetPosition.vi"("连接ID"=w459) -> ("y"=w454:dbl, "x"=w455:dbl, "连接ID 2"=w457:refnum<k5>, "c"=w451:dbl)  [unwired: 5 in]
                n239 = local write "RobAng"(w451) -> ()
                n240 = local write "机械手当前X坐标"(w455) -> ()
                n241 = local write "机械手当前Y坐标"(w454) -> ()
                n242 = Build Array (concatenate)(w456, w455, w454) -> (w453:dbl[])
                n243 = TCP Close Connection(connection ID=w457) -> ()  [unwired: 2 in, 2 out]
              }
              frame True {
                n244 = One Button Dialog(message="连接失败，请检查网络！" ("消息")) -> ()  [unwired: 1 in, 1 out]
              }
            }
          }
        }
        n245 = local write "操作状态"("示教基准位置" ("操作状态")) -> ()
        n246 = local write "相机三次采集"(TRUE ("机械手参数设置")) -> ()
      }
      frame "保存参数" {
        w479 = TRUE ("结束前等待")
        n247 = vi-ref "Caculator Save.vi"() -> (w478:refnum<vi>)
        n248 = local read "RobAng"() -> (w476:dbl)
        n249 = local write "操作状态"("保存参数" ("操作状态")) -> ()
        n250 = invoke class="VI" method="Ctrl Val.Set"(reference=w478, "Control Name"="RobAngle" ("控件名"), "Value"=w476) -> (reference out=w475:refnum<vi>)  [unwired: 2 in, 4 out]
        n251 = local read "CamAng"() -> (w472:dbl)
        n252 = invoke class="VI" method="Ctrl Val.Set"(reference=w475, "Control Name"="CamAngle" ("控件名"), "Value"=w472) -> (reference out=w473:refnum<vi>)  [unwired: 2 in, 4 out]
        n253 = invoke class="VI" method="Ctrl Val.Set"(reference=w473, "Control Name"="机械手" ("控件名"), "Value"=w484) -> (reference out=w483:refnum<vi>)  [unwired: 2 in, 4 out]
        n254 = local write "参数保存"(TRUE ("机械手参数设置")) -> ()
        n255 = local write "示教圆心"(TRUE ("机械手参数设置")) -> ()
        n256 = invoke class="VI" method="Ctrl Val.Set"(reference=w483, "Control Name"="像素" ("控件名"), "Value"=w480) -> (reference out=w482:refnum<vi>)  [unwired: 2 in, 4 out]
        n257 = invoke class="VI" method="FP.Open"(reference=w482, "Activate"=TRUE ("激活？"), "State"=T7."Standard" ("状态")) -> (reference out=w481:refnum<vi>)  [unwired: 2 in, 4 out]
        n258 = invoke class="VI" method="Run VI"(reference=w481, "Wait until done"=w479, "Auto Dispose Ref"=w479) -> ()  [unwired: 2 in, 5 out]
      }
      frame "完成" {
        n259 = local write "操作状态"("标定完成" ("操作状态")) -> ()
        n260 = control-ref of="本VI"() -> (w496:refnum<vi>)
        n261 = invoke class="VI" method="FP.Close"(reference=w496) -> ()  [unwired: 2 in, 3 out]
        n262 = call "自制光源控制.vi"("通道"=enum16{"CH1", "CH2", "CH3", "CH4"}."CH1", "VISA In"=refnum<visa-resource-name> "COM1", "错误输入"=w502, "操作模式"=enum16{"打开", "关闭", "设置"}."关闭", "baud rate"=u32 57600) -> ("错误输出"=w501:errorcluster)  [unwired: 4 in, 2 out]
      }
    }
    n263 = Wait (ms)(milliseconds to wait=u32 50 ("等待时间（毫秒）")) -> ()  [unwired: 1 out]
    n264 = local read "停止"() -> (w26:bool)
    n265 = Or(x=w27, y=w26) -> (x .or. y?=w25:bool)
  }
  "数组" <- w11
  "数组 2" <- w10
  n266 = while {
    stop <- w511 stop-if-true
    n267 = event shown="[0] 超时" {
      selector: _ -> [_ _]
      dyn-events: _ -> [_ _]
      timeout: 50 -> [_ _]
      tunnel: [_ w514] -> w512
      tunnel: [w513 _] -> w510
      event Timeout {
        n268 = event-data() -> ()  [unwired: 1 in, 3 out]
        n269 = local read "停止2"() -> (w513:bool)
      }
      event "强制退出": Value Change {
        n270 = event-data() -> ("NewVal"=w514:bool)  [unwired: 1 in, 5 out]
      }
    }
    n271 = local write "停止"(w512) -> ()
    n272 = Or(x=w512, y=w510) -> (x .or. y?=w511:bool)
  }
  n273 = local write "停止2"(w9) -> ()
  n274 = call <vilib>:"IMAQdx Close Camera.vi"("error in"=w15, "Session In"=w18) -> ()  [unwired: 9 in, 1 out]
  "停止" <- w8
  "停止2" <- w8
